vi "Stop Core.vi"(10 "final error code":i32, 11 "Study Actor in":refnum<class "Study Actor.lvclass">) -> (3 "Study Actor out":refnum<class "Study Actor.lvclass">)   [LabVIEW 2023, in "Study Actor.lvlib" / "Study Actor.lvclass"]
doc: "(<B>Filename</B>: Actor Framework.lvlib:Actor.lvclass:Stop Core.vi)\n\nDefines what the actor does before it stops. Use the <B>final error code</B> input to determine whether the actor shut down in response to an error.\n\nBy default, this method passes the Stop message along to all auto-stop nested actors. A descendant class may override this method to define additional behavior, such as shutting down any processes the actor initiated in its override of the Actor Core method."
uses:
  Study Actor.lvclass
  <vilib>/MGI/Panel Manager/Panel Actor/Panel Actor/Panel Actor.lvclass
  Study Actor.lvclass/Study Actor.ctl
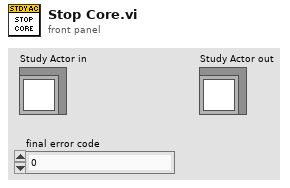
[diagram p1: front panel]
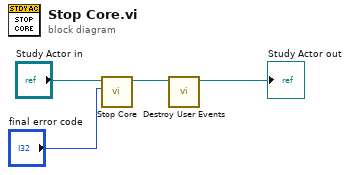
[diagram p0: block diagram]
diagram:
  n1 = call-parent "Stop Core.vi"("final error code"="final error code", "Actor in"="Study Actor in") -> ("Actor out"=w4:refnum<class "Study Actor.lvclass">)  [unwired: 9 in]
  n2 = call "Destroy User Events.vi"("Study Actor in"=w4) -> ("Study Actor out"=→"Study Actor out":refnum<class "Study Actor.lvclass">)  [unwired: 10 in]
